vi "get_element_at.vi"(6 "id chain":string[](array[string]), 7 "ignore IDs":bool, 8 "error in (no error)":errorcluster, 10 "key chain":string[](array[string]), 11 "Element in":refnum<class "XMLElement.lvclass">) -> (0 "error out":errorcluster, 1 "found?":bool, 2 "element":refnum<class "XMLElement.lvclass">, 3 "Element out":refnum<class "XMLElement.lvclass">)   [LabVIEW 2010, in "XMLElement.lvclass"]
uses:
  XMLElement.lvclass
  XMLElement.lvclass/XMLElement.ctl
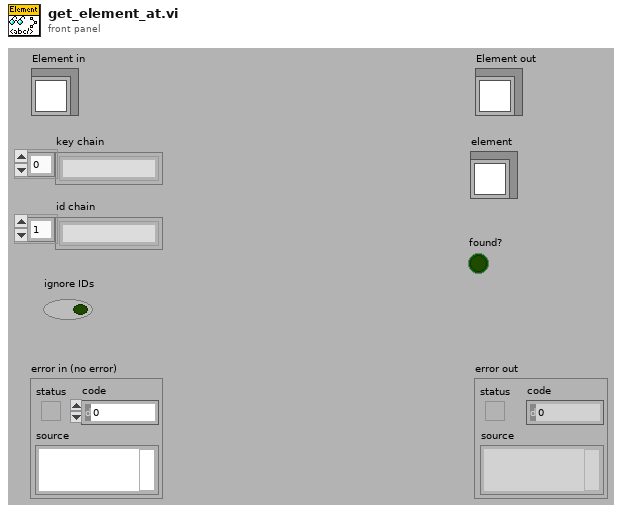
[diagram p1: front panel]
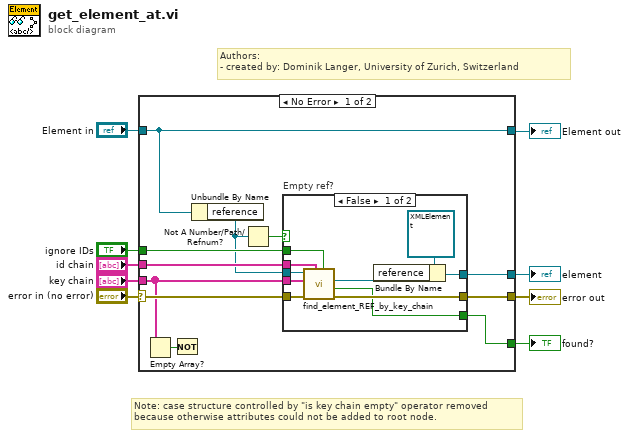
[diagram p0: block diagram]
diagram:
  # "Note: case structure controlled by \"is key chain empty\" operator removed\nbecause otherwise attributes could not be added to root node."
  # "Authors: \n- created by: Dominik Langer, University of Zurich, Switzerland"
  n1 = case shown="No Error" "error in (no error)" {
    selector: "error in (no error)" -> [w18 w33]
    tunnel: [w15 w33] -> w9
    tunnel: [w20 w32] -> w8
    tunnel: "Element in" -> [w20 w32]
    tunnel: "key chain" -> [w14 _]
    tunnel: "id chain" -> [w16 _]
    tunnel: [w19 _] -> w5
    tunnel: [w10 _] -> w4
    tunnel: "ignore IDs" -> [w17 _]
    frame No Error {
      n2 = Empty Array?(array=w14) -> (empty?=w11:bool)
      n3 = Not(x=w11) -> ()  [unwired: 1 out]
      n4 = Unbundle By Name(w20) -> ("reference"=w13:refnum<k20>)
      n5 = Not A Number/Path/Refnum?(number/path/refnum=w13) -> (NaN/Path/Refnum?=w12:bool)
      n6 = case "Empty ref?" shown="False" w12 {
        tunnel: [w29 _] -> w19
        tunnel: w14 -> [w28 _]
        tunnel: w18 -> [w27 w31]
        tunnel: w17 -> [w26 _]
        tunnel: w16 -> [w25 _]
        tunnel: [w24 w31] -> w15
        tunnel: [w22 _] -> w10
        tunnel: w13 -> [w21 _]
        frame False {
          n7 = call "find_element_REF_by_key_chain.vi"("ignore IDs"=w26, "id chain"=w25, "error in (no error)"=w27, "key chain"=w28, "element ref"=w21) -> ("error out"=w24:errorcluster, "found?"=w22:bool, "subelement ref"=w23:refnum<k20>)  [unwired: 4 in]
          n8 = Bundle By Name(cluster=refnum<class "XMLElement.lvclass"> refnum ("XMLElement.lvclass"), "reference"=w23) -> (w29:refnum<class "XMLElement.lvclass">)
        }
        frame True {
        }
      }
    }
    frame Error {
    }
  }
  "error out" <- w9
  "Element out" <- w8
  "element" <- w5
  "found?" <- w4
